vi "result judge double.vi"(9 "lower limit":dbl, 10 "upper limit":dbl, 11 "test value":dbl) -> (0 "pointValue":string, 1 "result string":string, 2 "result":bool)   [LabVIEW 2011]
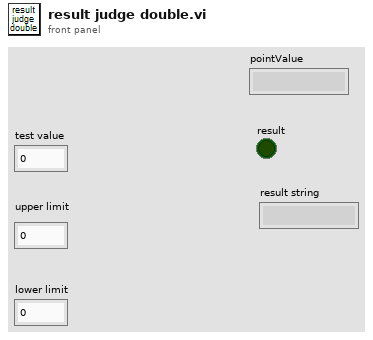
[diagram p1: front panel]
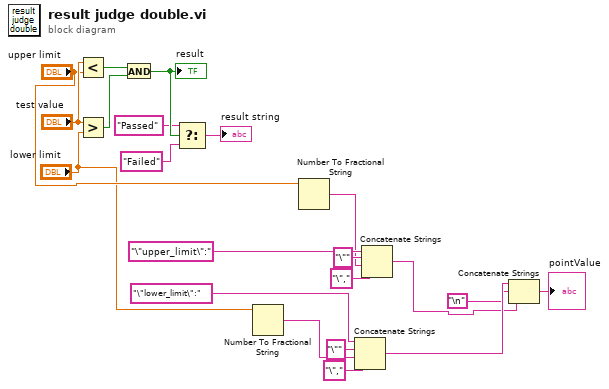
[diagram p0: block diagram]
diagram:
  n1 = Less?(x="test value", y="upper limit") -> (x < y?=w20:bool)
  n2 = Greater?(x="test value", y="lower limit") -> (0:w19:bool)
  n3 = And(x=w20, y=w19) -> (x .and. y?=w18:bool)
  "result" <- w18
  n4 = Select(t="Passed" ("TrueValue"), s=w18, f="Failed" ("FalseValue")) -> (s? t:f=→"result string":string)
  n5 = Number To Fractional String(number="lower limit") -> (F-format string=w5:string)  [unwired: 3 in]
  n6 = Number To Fractional String(number="upper limit") -> (F-format string=w10:string)  [unwired: 3 in]
  n7 = Concatenate Strings("\"lower_limit\":", "\"" ("字符串"), w5, "\"," ("字符串")) -> (w4:string)
  n8 = Concatenate Strings("\"upper_limit\":", "\"" ("字符串"), w10, "\"," ("字符串")) -> (w2:string)
  n9 = Concatenate Strings(w4, "\n", w2) -> (→"pointValue":string)
